vi "math.vi"(9 "input":i32) -> (2 "output":dbl)   [LabVIEW 2013]
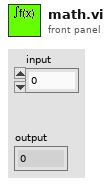
[diagram p1: front panel]
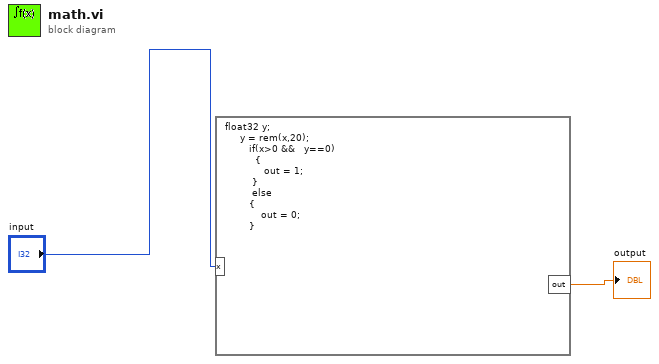
[diagram p0: block diagram]
diagram:
  n1 = formula code="float32 y;\n     y = rem(x,20);\n        if(x>0 &&   y==0)\n          {\n             out = 1;\n         }\n         else \n        {\n            out = 0;\n        }"("x"="input") -> ("out"=→"output":dbl)
